vi "niRFUtil MEAS Origin Offset.vi"(0 "Waveform In":T1 {"y" format="%.2f"; "dx" format="%^.2e"; "x0" format="%^.2e"}, 1 "Frequency Offset (Hz)":sgl format="%^.2e", 2 "Initial Phase (deg)":sgl format="%.2f", 5 "Reference Waveform In":T1 {"y" format="%.2f"; "dx" format="%^.2e"; "x0" format="%^.2e"}, 7 "Correct Phase/Frequency Offset?":bool, 9 "Threshold?":bool, 12 "Origin Offset Threshold (dBm)":sgl=inf, 13 "Compute Gain?":bool) -> (4 "Gain (dB)":sgl, 6 "Gain (linear)":sgl, 8 "Origin Offset":csg format="%#.4g", 10 "Origin Offset (dB)":sgl)   [LabVIEW 2015, in "niRFUtil.lvlib"]
uses:
  niRFUtil.lvlib
  Includes/niRFUtil INC Complex Waveform.ctl
  Includes/niRFUtil INC Complex Array.ctl
  Conversion/niRFUtil CONV dBm to 1 Ohm Voltage (real scalar).vi
  niRFUtil MEAS Mean (real array).vi
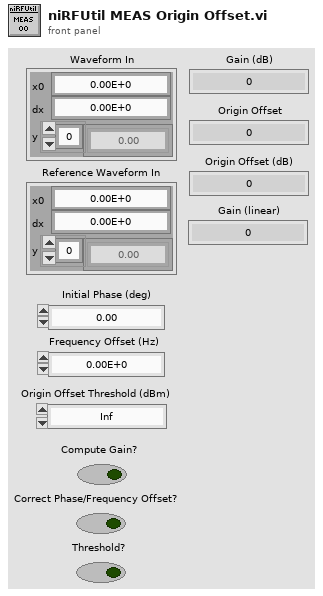
[diagram p1: front panel]
types:
  T1 = typedef "niRFUtil.lvlib/niRFUtil INC Complex Waveform.ctl" = cluster{"x0":dbl, "dx":dbl, "y":T2}
  T2 = typedef "niRFUtil.lvlib/niRFUtil INC Complex Array.ctl" = csg[]
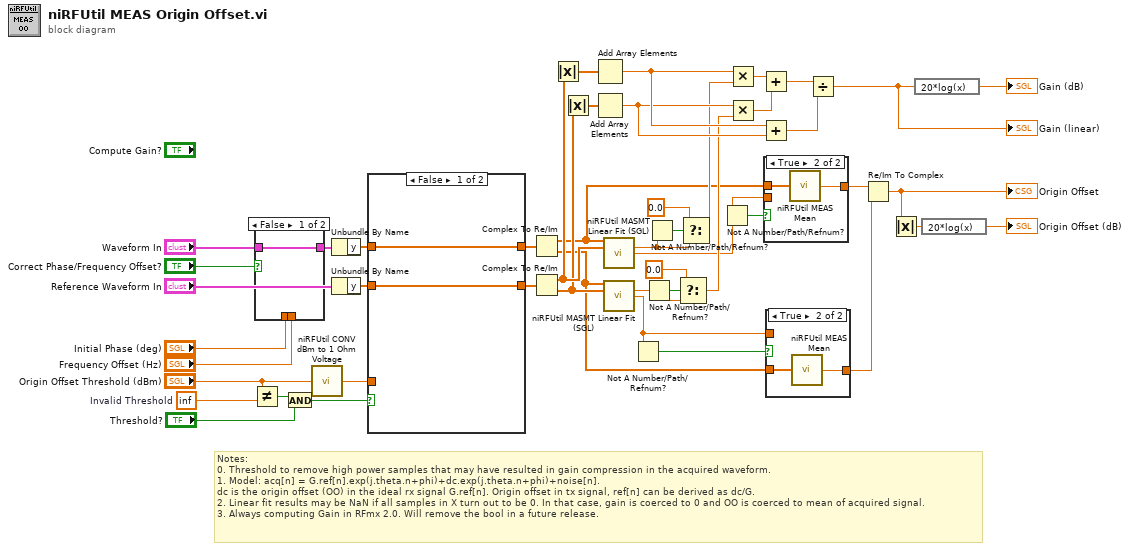
[diagram p0: block diagram]
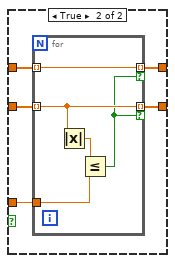
[diagram p4: hidden frame]
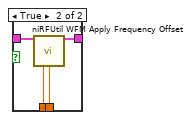
[diagram p5: hidden frame]
diagram:
  w29 = sgl inf  # Invalid Threshold
  # "Notes:\n0. Threshold to remove high power samples that may have resulted in gain compression in the acquired waveform.\n1. Model: acq[n] = G.ref[n].exp(j.theta.n+phi)+dc.exp(j.theta.n+phi)+noise[n]. \ndc is the origin offset (OO) in the ideal rx signal G.ref[n]. Origin offset in tx signal, ref[n] can be derived as dc/G.\n2. Linear fit results may be NaN if all samples in X turn out to be 0. In that case, gain is coerced to 0 and OO is coerced to mean of acquired signal.\n3. Always computing Gain in RFmx 2.0. Will remove the bool in a future release."
  n1 = Not Equal?(x="Origin Offset Threshold (dBm)", y=w29) -> (x != y?=w28:bool)
  n2 = case shown="False" "Correct Phase/Frequency Offset?" {
    tunnel: "Waveform In" -> [w48 w52]
    tunnel: [w48 w51] -> w31
    tunnel: "Initial Phase (deg)" -> [_ w50]
    tunnel: "Frequency Offset (Hz)" -> [_ w49]
    frame False {
    }
    frame True {
      n3 = call "niRFUtil WFM Apply Frequency Offset.vi"("Waveform In"=w52, "Initial Phase (deg)"=w50, "Offset (Hz)"=w49) -> ("Waveform Out"=w51:T1)  [unwired: 11 in, 1 out]
    }
  }
  n4 = And(x=w28, y="Threshold?") -> (x .and. y?=w26:bool)
  n5 = call-poly "niRFUtil CONV dBm to 1 Ohm Voltage.vi"("Real Scalar (dBm)"="Origin Offset Threshold (dBm)") -> ("Real Scalar (V)"=w34:sgl)  [unwired: 14 in]
  n6 = Unbundle By Name(w31) -> ("y"=w37:T2)
  n7 = Unbundle By Name("Reference Waveform In") -> ("y"=w35:T2)
  n8 = case shown="False" w26 {
    tunnel: [w54 w59] -> w38
    tunnel: w37 -> [w54 w58]
    tunnel: [w53 w57] -> w36
    tunnel: w35 -> [w53 w56]
    tunnel: w34 -> [_ w55]
    frame False {
    }
    frame True {
      n9 = for {
        tunnel: [w64] -> w59 mode=indexing if=w60
        tunnel: w58 -> [w64] mode=indexing
        tunnel: [w63] -> w57 mode=indexing if=w60
        tunnel: w56 -> [w63] mode=indexing
        tunnel: w55 -> [w61]
        n10 = Absolute Value(x=w63) -> (abs(x)=w62:sgl)
        n11 = Less Or Equal?(x=w62, y=w61) -> (x <= y?=w60:bool)
      }
    }
  }
  n12 = Complex To Re/Im(x + iy=w38) -> (x=w3:sgl[], y=w11:sgl[])
  n13 = Complex To Re/Im(x + iy=w36) -> (x=w33:sgl[], y=w32:sgl[])
  n14 = Absolute Value(x=w33) -> (abs(x)=w25:sgl[])
  n15 = Absolute Value(x=w32) -> (abs(x)=w24:sgl[])
  n16 = Add Array Elements(numeric array=w25) -> (sum=w20:sgl)
  n17 = Add Array Elements(numeric array=w24) -> (sum=w19:sgl)
  n18 = call "niRFUtil MASMT Linear Fit (SGL).vi"("Y"=w3, "X"=w33) -> ("slope"=w6:sgl, "intercept"=w2:sgl)  [unwired: 9 in, 3 out]
  n19 = call "niRFUtil MASMT Linear Fit (SGL).vi"("Y"=w11, "X"=w32) -> ("slope"=w15:sgl, "intercept"=w9:sgl)  [unwired: 9 in, 3 out]
  n20 = Not A Number/Path/Refnum?(number/path/refnum=w9) -> (NaN/Path/Refnum?=w12:bool)
  n21 = Not A Number/Path/Refnum?(number/path/refnum=w15) -> (NaN/Path/Refnum?=w16:bool)
  n22 = Not A Number/Path/Refnum?(number/path/refnum=w6) -> (NaN/Path/Refnum?=w7:bool)
  n23 = Select(t=sgl 0.0, s=w16, f=w15) -> (s? t:f=w14:sgl)
  n24 = Select(t=sgl 0.0, s=w7, f=w6) -> (s? t:f=w5:sgl)
  n25 = Not A Number/Path/Refnum?(number/path/refnum=w2) -> (NaN/Path/Refnum?=w4:bool)
  n26 = Multiply(x=w20, y=w5) -> (x*y=w23:sgl)
  n27 = Multiply(x=w19, y=w14) -> (x*y=w22:sgl)
  n28 = Add(x=w23, y=w22) -> (x+y=w21:sgl)
  n29 = Add(x=w20, y=w19) -> (x+y=w18:sgl)
  n30 = case shown="True" w4 {
    tunnel: w3 -> [_ w67]
    tunnel: [w65 w66] -> w1
    tunnel: w2 -> [w65 _]
    frame False {
    }
    frame True {
      n31 = call-poly "niRFUtil MEAS Mean.vi"("Real Array"=w67) -> ("Mean"=w66:sgl)  [unwired: 14 in]
    }
  }
  n32 = case shown="True" w12 {
    tunnel: w11 -> [_ w70]
    tunnel: [w68 w69] -> w10
    tunnel: w9 -> [w68 _]
    frame False {
    }
    frame True {
      n33 = call-poly "niRFUtil MEAS Mean.vi"("Real Array"=w70) -> ("Mean"=w69:sgl)  [unwired: 14 in]
    }
  }
  n34 = Divide(x=w21, y=w18) -> (x/y=w17:sgl)
  "Gain (linear)" <- w17
  n35 = Re/Im To Complex(1:w10, 2:w1) -> (0:w44:csg)
  "Origin Offset" <- w44
  n36 = Absolute Value(x=w44) -> (abs(x)=w45:sgl)
  n37 = expression code="20*log(x)"(w17) -> (→"Gain (dB)":sgl)
  n38 = expression code="20*log(x)"(w45) -> (→"Origin Offset (dB)":sgl)
